vi "RT Driver VI_InlineAsync.vi"(7 "Operation":T1(ring), 11 "Device Reference in":u64 format="%.0x") -> (0 "Error Code":i32)   [LabVIEW 2026]
uses:
  VS Custom Device API/VS Custom Device API.lvclass
  C:/dev/cd20_main/Source/niveristand-custom-device-wizard/ProjectTemplate/Source/NI VeriStand/Custom Device Express/Custom Device/Template Files/Engine/VS Custom Device API/VS Custom Device API.lvclass
  C:/Program Files/NI/LVAddons/nivscustomdeviceexpress/1/Targets/win64/user.lib/CustomDeviceInterfaces_v1.lvlibp/custom-device-express-framework/Source/Custom Device Interfaces/CustomDeviceAPI/CustomDeviceAPI.lvclass
  Template Engine.lvlib
  <userlib>/CustomDeviceInterfaces_v1.lvlibp/custom-device-express-framework/Source/Custom Device Interfaces/Utility/CustomDeviceUtility.lvclass
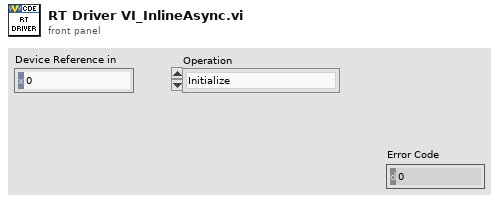
[diagram p1: front panel]
types:
  T1 = enum16{"Initialize", "Start", "Read Data from HW", "Write Data to HW", "Close"}
  T2 = cluster{"CDUtility":refnum<class "CustomDeviceUtility.lvclass">, "VS Engine CDAPI":refnum<class "VS Custom Device API.lvclass">}
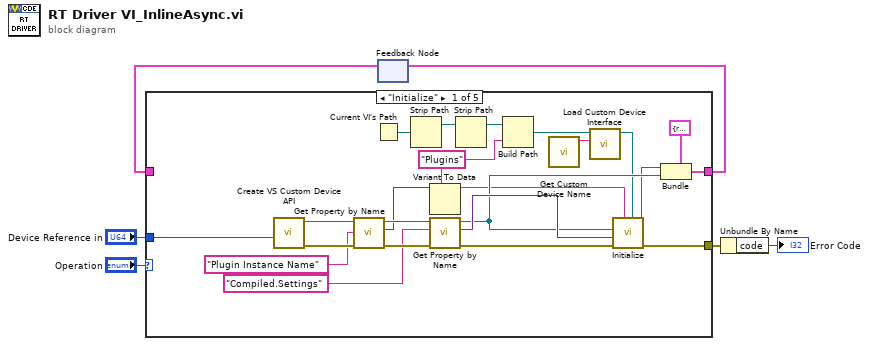
[diagram p0: block diagram]
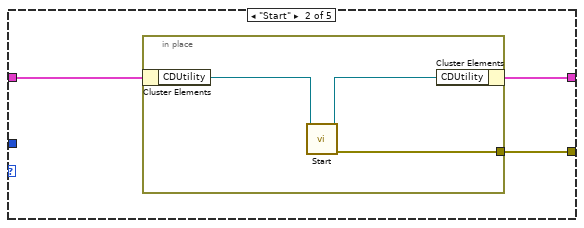
[diagram p2: hidden frame]
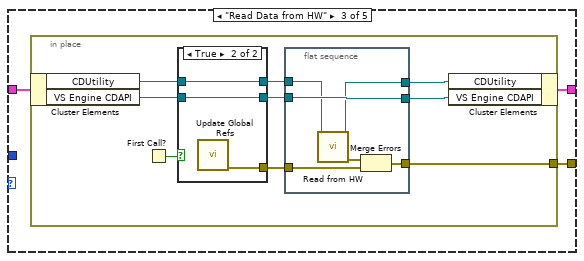
[diagram p3: hidden frame]
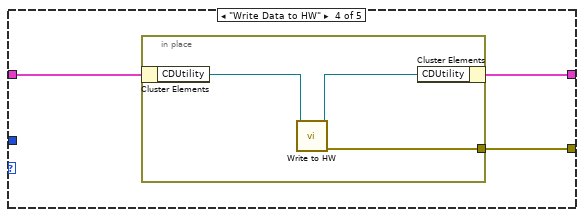
[diagram p5: hidden frame]
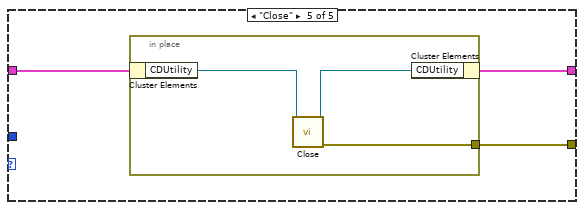
[diagram p6: hidden frame]
diagram:
  n1 = feedback #1() -> (w3:T2)  [unwired: 1 in]
  n2 = case shown="\"Initialize\"" "Operation" {
    tunnel: [w9 w31 w36 w59 w65] -> w4
    tunnel: w3 -> [_ w30 w37 w60 w66]
    tunnel: "Device Reference in" -> [w21 _ _ _ _]
    tunnel: [w26 w32 w38 w61 w67] -> w6
    frame "Initialize" {
      w7 = "Plugins" ("Plugin Name")
      n3 = call "Create VS Custom Device API.vi"("Custom Device Item Ref"=w21) -> ("error out"=w27:errorcluster, "VS CDAPI out"=w25:refnum<class "VS Custom Device API.lvclass">)  [unwired: 9 in]
      n4 = call-dynamic "Get Property by Name.vi"("error in"=w27, "Property Name"="Plugin Instance Name", "VS CD API in"=w25) -> ("error out"=w29:errorcluster, "Value"=w23:variant, "VS CDAPI out"=w24:refnum<class "VS Custom Device API.lvclass">)  [unwired: 6 in]
      n5 = Current VI's Path() -> (path=w15:path)
      n6 = Strip Path(path=w15) -> (stripped path=w14:path)  [unwired: 1 out]
      n7 = Variant To Data(type=w7, Variant=w23) -> (data=w16:string)  [unwired: 1 in, 1 out]
      n8 = call-dynamic "Get Property by Name.vi"("error in"=w29, "Property Name"="Compiled.Settings", "VS CD API in"=w24) -> ("error out"=w28:errorcluster, "Value"=w22:variant, "VS CDAPI out"=w20:refnum<class "VS Custom Device API.lvclass">)  [unwired: 6 in]
      n9 = Strip Path(path=w14) -> (stripped path=w13:path)  [unwired: 1 out]
      n10 = Build Path(base path=w13, name or relative path=w7) -> (appended path=w12:path)
      n11 = call "Get Custom Device Name.vi"() -> ("CD Name"=w8:string)  [unwired: 11 in]
      n12 = call <userlib>:"Load Custom Device Interface.vi"("Plugin Name"=w8, "Path"=w12) -> ("iCD out"=w17:refnum<class "CustomDevice.lvclass">)  [unwired: 8 in, 1 out]
      n13 = call <userlib>:"Initialize.vi"("iCD in"=w17, "Custom Device Name"=w16, "error in"=w28, "Compiled Settings"=w22, "iCDAPI in"=w20) -> ("error out"=w26:errorcluster, "Utlity out"=w10:refnum<class "CustomDeviceUtility.lvclass">)  [unwired: 5 in]
      n14 = Bundle(cluster=T2 {"CDUtility"=refnum, "VS Engine CDAPI"=refnum}, "CDUtility"=w10, "VS Engine CDAPI"=w20) -> (w9:T2)
    }
    frame "Start" {
      n15 = in-place {
        in-place-border: [w35] -> w32
        n16 = in-place-cluster #2(w30) -> ("CDUtility"=w34:refnum<class "CustomDeviceUtility.lvclass">)
        n17 = call <userlib>:"Start.vi"("Utility in"=w34) -> ("error out"=w35:errorcluster, "Utility out"=w33:refnum<class "CustomDeviceUtility.lvclass">)  [unwired: 9 in]
        n18 = in-place-cluster #2("CDUtility"=w33) -> (w31:T2)
      }
    }
    frame "Read Data from HW" {
      n19 = in-place {
        in-place-border: [w47] -> w38
        n20 = in-place-cluster #3(w37) -> ("CDUtility"=w43:refnum<class "CustomDeviceUtility.lvclass">, "VS Engine CDAPI"=w44:refnum<class "VS Custom Device API.lvclass">)
        n21 = First Call?() -> (First Call?: T/F=w45:bool)
        n22 = case shown="True" w45 {
          tunnel: [_ w58] -> w46
          tunnel: w44 -> [w55 w57]
          tunnel: [w55 w57] -> w40
          tunnel: w43 -> [w54 w56]
          tunnel: [w54 w56] -> w42
          frame False {
          }
          frame True {
            n23 = call "Update Global Refs.vi"() -> ("error out"=w58:errorcluster)  [unwired: 11 in]
          }
        }
        n24 = flat-sequence {
          tunnel: [w52] -> w47
          tunnel: w46 -> [w51]
          tunnel: w42 -> [w48]
          tunnel: [w49] -> w41
          tunnel: w40 -> [w50]
          tunnel: [w50] -> w39
          frame #0 {
            n25 = call <userlib>:"Read from HW.vi"("Utility in"=w48) -> ("error out"=w53:errorcluster, "Utility out"=w49:refnum<class "CustomDeviceUtility.lvclass">)  [unwired: 9 in]
            n26 = Merge Errors(w53, w51) -> (w52:errorcluster)
          }
        }
        n27 = in-place-cluster #3("CDUtility"=w41, "VS Engine CDAPI"=w39) -> (w36:T2)
      }
    }
    frame "Write Data to HW" {
      n28 = in-place {
        in-place-border: [w64] -> w61
        n29 = in-place-cluster #4(w60) -> ("CDUtility"=w63:refnum<class "CustomDeviceUtility.lvclass">)
        n30 = call <userlib>:"Write to HW.vi"("Utility in"=w63) -> ("error out"=w64:errorcluster, "Utility out"=w62:refnum<class "CustomDeviceUtility.lvclass">)  [unwired: 9 in]
        n31 = in-place-cluster #4("CDUtility"=w62) -> (w59:T2)
      }
    }
    frame "Close" {
      n32 = in-place {
        in-place-border: [w70] -> w67
        n33 = in-place-cluster #5(w66) -> ("CDUtility"=w69:refnum<class "CustomDeviceUtility.lvclass">)
        n34 = call <userlib>:"Close.vi"("Utility in"=w69) -> ("error out"=w70:errorcluster, "Utility out"=w68:refnum<class "CustomDeviceUtility.lvclass">)  [unwired: 9 in]
        n35 = in-place-cluster #5("CDUtility"=w68) -> (w65:T2)
      }
    }
  }
  n36 = feedback-in #1(w4) -> ()
  n37 = Unbundle By Name(w6) -> ("code"=→"Error Code":i32)
